vi "Multiply.vi"() -> ()   [LabVIEW 2017]
panel:
  out "C":i32
  in  "B":i32
  in  "A":i32
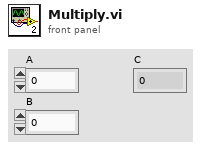
[diagram p1: front panel]
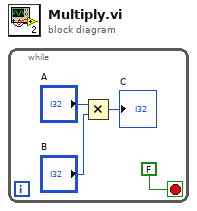
[diagram p0: block diagram]
diagram:
  n1 = while {
    stop <- FALSE stop-if-true
    n2 = Multiply(x="A", y="B") -> (x*y=→"C":i32)
  }
